vi "PyListToStringvi.vi"(1 "PythonList":string) -> (0 "String":string)   [LabVIEW 2014]
panel:
  # "items are deliminted by \""
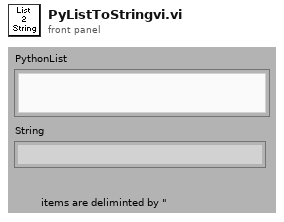
[diagram p1: front panel]
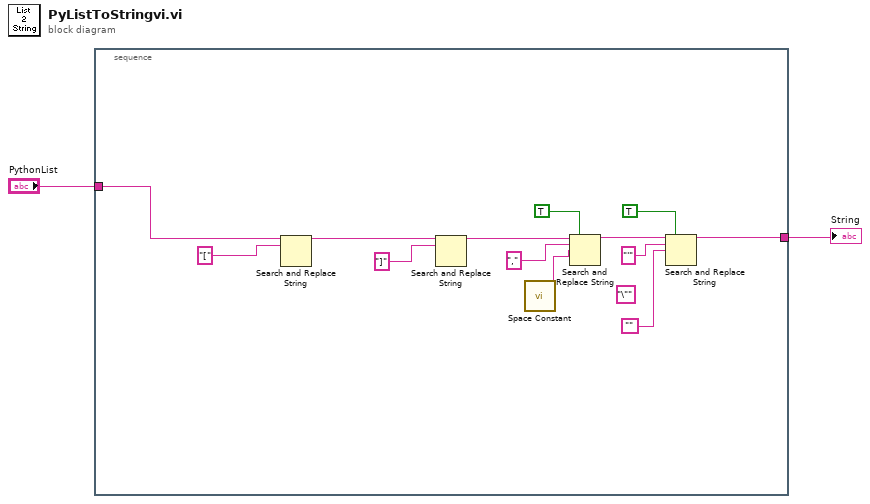
[diagram p0: block diagram]
diagram:
  n1 = stacked-sequence {
    tunnel: "PythonList" -> [w15]
    tunnel: [w7] -> w1
    frame #0 {
      (unwired) "\"" ("search string")
      n2 = Search and Replace String(input string=w15, search string="[") -> (result string=w12:string)  [unwired: 6 in, 3 out]
      n3 = Search and Replace String(input string=w12, search string="]") -> (result string=w10:string)  [unwired: 6 in, 3 out]
      n4 = call <vilib>:"Space Constant.vi"() -> ("String"=w9:string)
      n5 = Search and Replace String(replace all?=TRUE ("replace all? (F)"), input string=w10, search string=",", replace string=w9) -> (result string=w8:string)  [unwired: 4 in, 3 out]
      n6 = Search and Replace String(replace all?=TRUE ("replace all? (F)"), input string=w8, search string="'", replace string="") -> (result string=w7:string)  [unwired: 4 in, 3 out]
    }
  }
  "String" <- w1
